vi "Mux4Way16.vi"(1 "sel":bool[](array[boolean]), 3 "d":bool[](array[boolean]), 4 "c":bool[](array[boolean]), 5 "b":bool[](array[boolean]), 6 "a":bool[](array[boolean])) -> (0 "out":bool[](array[boolean]))   [LabVIEW 2014]
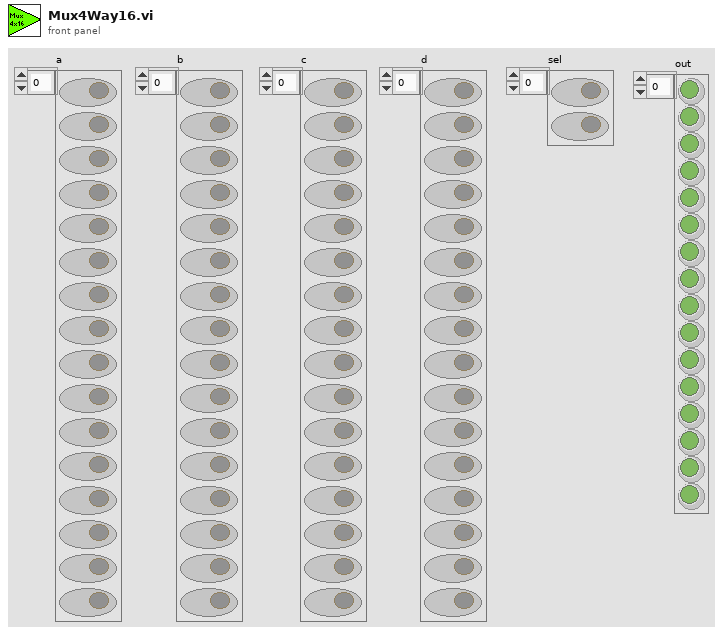
[diagram p1: front panel]
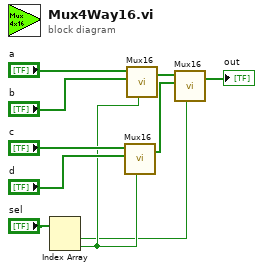
[diagram p0: block diagram]
diagram:
  n1 = Index Array(array="sel") -> (element #1=w1:bool, element #2=w5:bool)  [unwired: 2 in]
  n2 = call "Mux16.vi"("sel"=w5, "b"="d", "a"="c") -> ("out"=w3:bool[])  [unwired: 4 in]
  n3 = call "Mux16.vi"("sel"=w5, "b"="b", "a"="a") -> ("out"=w4:bool[])  [unwired: 4 in]
  n4 = call "Mux16.vi"("sel"=w1, "b"=w3, "a"=w4) -> ("out"=→"out":bool[])  [unwired: 4 in]
